vi "VI-Replace Events on State Cluster.vi"(0 "XCtl Path in":path, 11 "error in (no error)":errorcluster, 12 "Event Data typedef":path) -> (4 "XCtl Path out":path, 15 "error out":errorcluster)   [LabVIEW 2015]
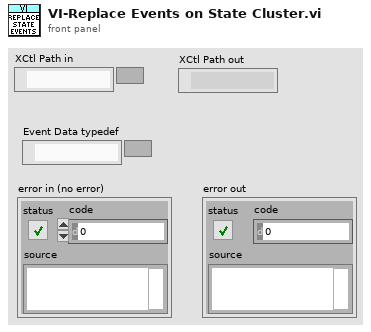
[diagram p1: front panel]
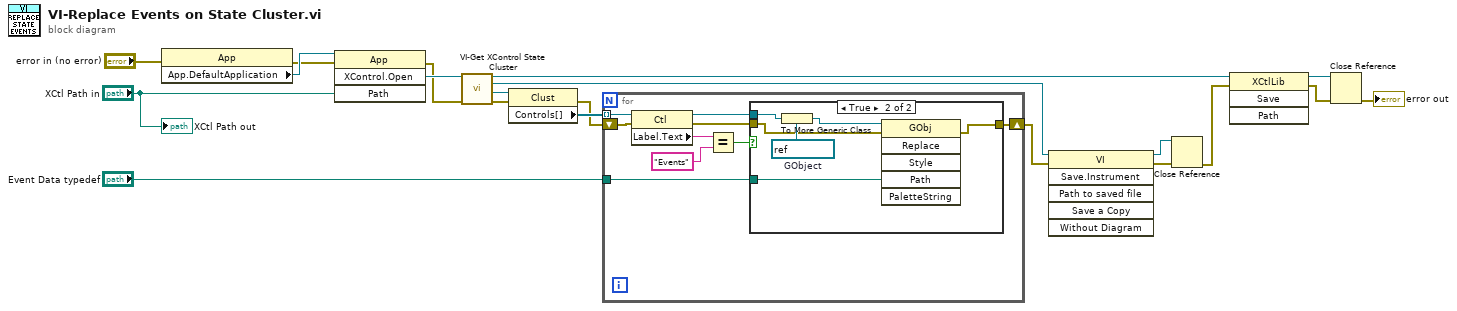
[diagram p0: block diagram]
diagram:
  n1 = property class="App"(error in="error in (no error)") -> (error out=w16:errorcluster, "App.DefaultApplication"=w17:refnum<vi>)  [unwired: 1 in, 1 out]
  n2 = invoke class="App" method="XControl.Open"(reference=w17, error in=w16, "Path"="XCtl Path in") -> (error out=w7:errorcluster, "Open XControl"=w13:refnum<vi>)  [unwired: 1 in, 2 out]
  n3 = call "VI-Get XControl State Cluster.vi"("XControlLibrary in"=w13, "error in (no error)"=w7) -> ("XControlLibrary out"=w8:refnum<vi>, "VI ref"=w18:refnum<vi>, "State cluster"=w5:refnum<vi>, "error out"=w6:errorcluster)  [unwired: 10 in]
  n4 = property class="Clust"(reference=w5, error in=w6) -> (error out=w3:errorcluster, "Controls[]"=w4:refnum<vi>[])  [unwired: 1 out]
  n5 = for {
    tunnel: w4 -> [w29] mode=indexing
    shift-right: [w21] -> w1
    shift-left: w3 -> [w28]
    tunnel: "Event Data typedef" -> [w22]
    n6 = property class="Ctl"(reference=w29, error in=w28) -> (reference out=w23:refnum<vi>, error out=w24:errorcluster, "Label.Text"=w27:string)
    n7 = Equal?(x=w27, y="Events") -> (x = y?=w25:bool)
    n8 = case shown="True" w25 {
      tunnel: w24 -> [w30 w33]
      tunnel: w23 -> [_ w36]
      tunnel: w22 -> [_ w32]
      tunnel: [w30 w31] -> w21
      frame False {
      }
      frame True {
        w35 = refnum<vi> refnum  # GObject
        n9 = To More Generic Class(target class=w35, reference=w36) -> (generic class reference=w34:refnum<vi>)
        n10 = invoke class="GObj" method="Replace"(reference=w34, error in=w33, "Path"=w32) -> (error out=w31:errorcluster)  [unwired: 3 in, 5 out]
      }
    }
  }
  n11 = invoke class="VI" method="Save.Instrument"(reference=w18, error in=w1) -> (reference out=w20:refnum<vi>, error out=w19:errorcluster)  [unwired: 4 in, 4 out]
  n12 = Close Reference(reference=w20, error in (no error)=w19) -> (error out=w10:errorcluster)
  n13 = invoke class="XCtlLib" method="Save"(reference=w8, error in=w10) -> (reference out=w11:refnum<vi>, error out=w12:errorcluster)  [unwired: 2 in, 2 out]
  n14 = Close Reference(reference=w11, error in (no error)=w12) -> (error out=→"error out":errorcluster)
  "XCtl Path out" <- "XCtl Path in"
